vi "CAL-Probe Tube Cal Path (L-R).vi"(0 "Ear":T1, 5 "Probe Tube Folder":path=path "C:/Data/Probe Tube Calibrations", 7 "Right":string, 9 "Left":string, 11 "error in (no error)":errorcluster) -> (6 "Probe Tube Cal Path":path, 15 "error out":errorcluster)   [LabVIEW 2020]
uses:
  epl-vi-lib/Utility VIs/Type Defs/Left-Right ring.ctl
  SubVIs/Calibration Globals.vi
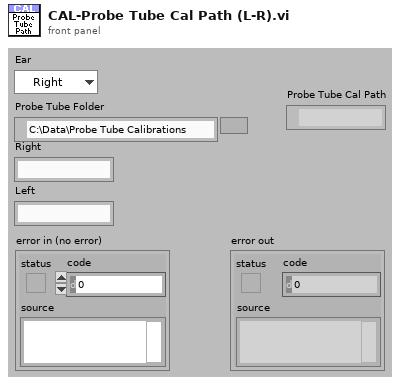
[diagram p1: front panel]
types:
  T1 = typedef "Left-Right ring.ctl" = enum16{"Right", "Left"}
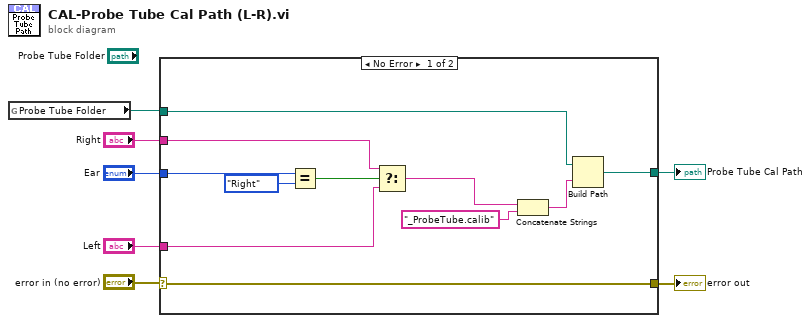
[diagram p0: block diagram]
diagram:
  n1 = global read "Calibration Globals.vi" "Probe Tube Folder"() -> (w1:path)
  n2 = case shown="No Error" "error in (no error)" {
    selector: "error in (no error)" -> [w10 w19]
    tunnel: "Ear" -> [w18 _]
    tunnel: "Right" -> [w17 _]
    tunnel: "Left" -> [w16 _]
    tunnel: w1 -> [w13 _]
    tunnel: [w11 _] -> w3
    tunnel: [w10 w19] -> w2
    frame No Error {
      n3 = Equal?(x=w18, y=Left-Right_ring."Right") -> (x = y?=w8:bool)
      n4 = Select(t=w17, s=w8, f=w16) -> (s? t:f=w14:string)
      n5 = Concatenate Strings(w14, "_ProbeTube.calib" ("string")) -> (w12:string)
      n6 = Build Path(base path=w13, name or relative path=w12) -> (appended path=w11:path)
    }
    frame Error {
    }
  }
  "error out" <- w2
  "Probe Tube Cal Path" <- w3
